vi "zlgcan_demo_CANFDNET_UDP.vi"() -> ()   [LabVIEW 2018]
doc: "适用的设备：CANET-E-U、CANET-2E-U、CANET-4E-U、CANET-8E-U、\nCANET-200T、CANET-100T"
uses:
  zlgcan_demo_CANFDNET_UDP/bin/zlgcan.dll
  zlgcan_demo_CANFDNET_UDP/bin/zlgcan_wrap.dll
  data_type/ZCAN_TransmitFD_Data.ctl
  data_type/ZCAN_Transmit_Data.ctl
panel:
  in  "ZCAN_Transmit_Data":T1
  in  "ZCAN_TransmitFD_Data":T2
  in  "CANFD数据帧数组":T3(array[cluster])
  in  "CAN数据帧数组":T4(array[cluster])
  out "已接收帧数":u32
  out "CAN报文显示":string[][](table)
  out "CANFD报文显示":string[][](table)
  out "error out 2":errorcluster caption="错误输出"
  out "source":string
  in  "开启CAN":bool
  in  "stop":bool
  in  "?":T5(tab)
  in  "CAN卡型号":u32(ring)=49 items=["CANFDNET_800U_UDP"=58, "CANFDNET_400U_UDP"=53, "CANFDNET_100U_UDP"=56, "CANFDNET-200U-UDP"=49]
  in  "索引":u32(ring) items=["0", "1", "2", "3", "4", "5", "6", "7", "8"]
  in  "CAN 通道":u32(ring) items=["0", "1", "2", "3"]
  out "设备句柄":u32
  out "通道句柄":u32
  out "error out":errorcluster caption="状态"
  in  "发送":bool
  in  "ID":u32=18 format="0x%08x"
  in  "帧类型":u32(ring) items=["标准帧", "扩展帧"]
  in  "帧格式":u32(ring) items=["数据帧", "远程帧"]
  in  "发送方式":u32(ring) items=["正常发送", "单次发送", "自发自收", "单次自发自收"]
  in  "协议":u32(ring) items=["CAN", "CANFD"]
  in  "数据输入":string="11 22 33 44 55 66 77 88"
  in  "CANFD加速？":u32(ring) items=["不加速", "加速"]
  out "数据长度":u8=8 max=8
  # "适用的设备：CANFDNET-100U-UDP、CANFDNET-200U-UDP、CANFDNET-400U-UDP、CANFDNET-800U-UDP"
  # "参数设置这里的参数需要到后面板进行设置"
  # "停止程序前，\n请先关闭CAN卡"
  # "当CANFDNET的工作模式为：\n\n1. 客户端（TCP Client）\n\n   LabVIEW 设备型号选择【 CANFDNET-TCP】\n\n   TCP模式选择【服务器 TCP Sever】\n\n   填写电脑本机IP+本地端口。\n\n2. 服务器（TCP Sever）\n\n   LabVIEW 设备型号选择【 CANFDNET-TCP】\n\n   TCP模式选择【客户端 TCP Client】\n\n   填写CANFDNET的 IP +工作端口\n\n3. UDP\n\n   LabVIEW 设备型号选择【 CANFDNET-UDP】\n\n   填写CANFDNET的IP+工作端口+本地端口"
  # "1. 调试运行DEMO前，将bin文件夹下面的kerneldlls文件夹先拷贝至LabView安装目录，\n如 D:\\Program Files (x86)\\National Instruments\\LabVIEW 2018。"
  # "2. 确保电脑有VC++ 2005/2008/2010/2013运行库（对应32，64位），可到微软官网下载。"
  # "3，如果打开设备失败，可能原因：\n（1）没有进行第二步操作；\n（2）已经打开过一次，没有正常关闭的情况下，继续点击“打开设备”，是无法打开的。\n     需要USB重新拔插，LABVIEW重启（全部关闭），然后再“打开设备”。\n (3) 项目路径不能有中文繁体。"
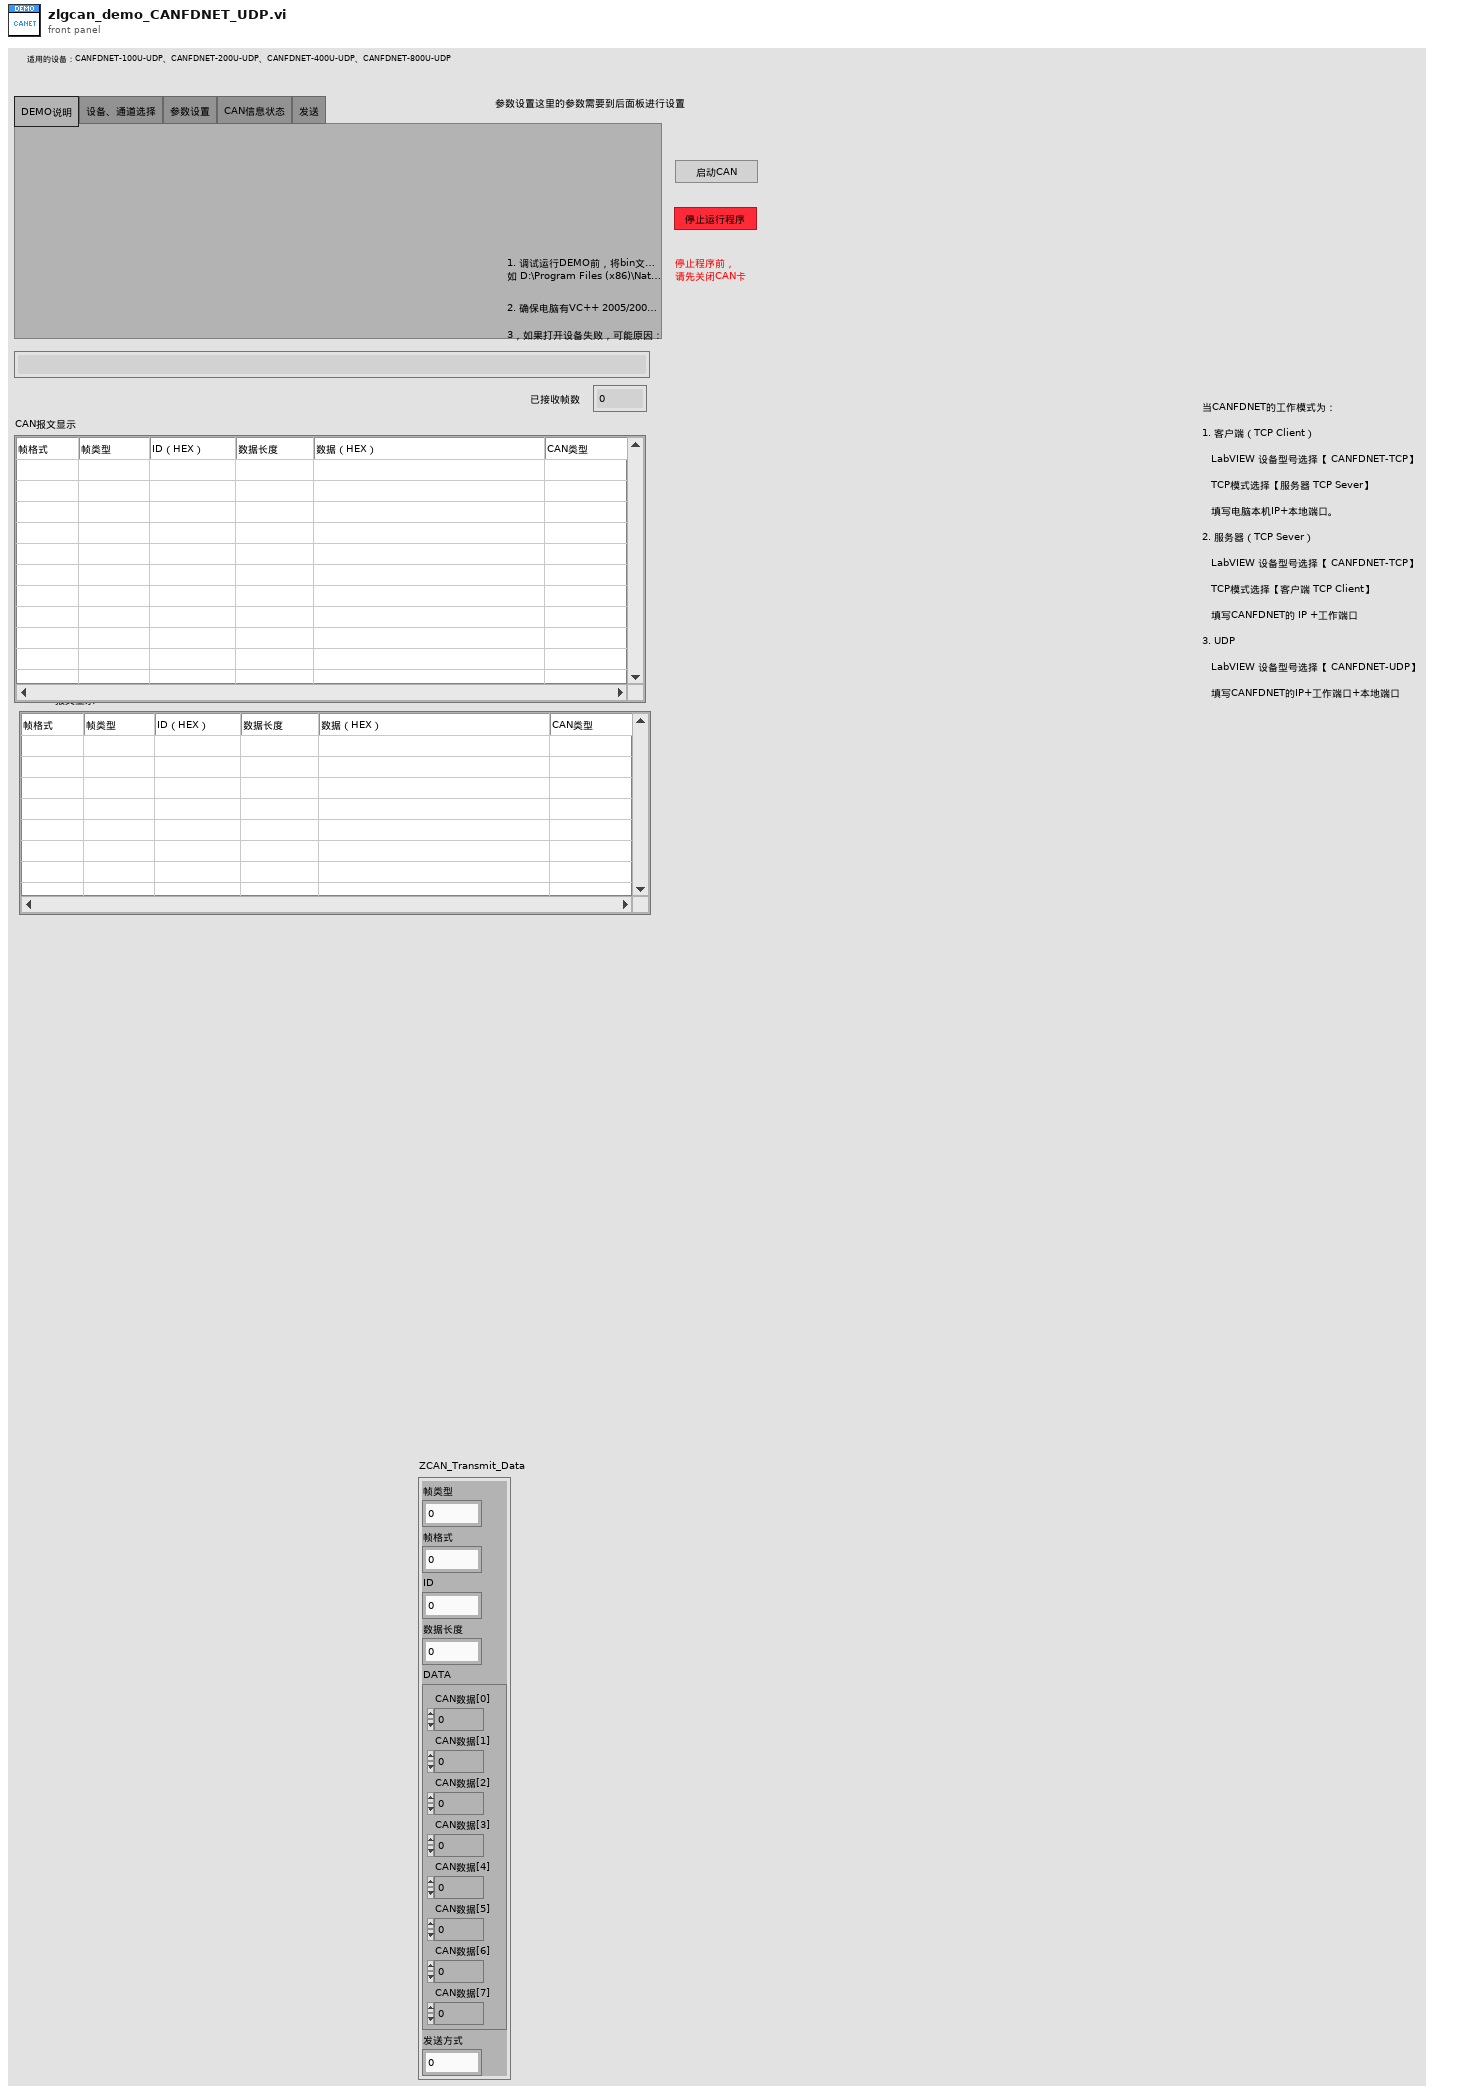
[diagram p1: front panel]
types:
  T1 = typedef "ZCAN_Transmit_Data.ctl" = cluster{"帧类型":u32, "帧格式":u32, "ID":u32, "数据长度":u8, "DATA":cluster{"CAN数据[0]":u8, "CAN数据[1]":u8, "CAN数据[2]":u8, "CAN数据[3]":u8, "CAN数据[4]":u8, "CAN数据[5]":u8, "CAN数据[6]":u8, "CAN数据[7]":u8}, "发送方式":u32}
  T2 = typedef "ZCAN_TransmitFD_Data.ctl" = cluster{"帧类型":u32, "帧格式":u32, "ID":u32, "数据长度":u8, "CANFD加速？":u8, "DATA":cluster{"CAN数据[0]":u8, "CAN数据[1]":u8, "CAN数据[2]":u8, "CAN数据[3]":u8, "CAN数据[4]":u8, "CAN数据[5]":u8, "CAN数据[6]":u8, "CAN数据[7]":u8, "CAN数据[8]":u8, "CAN数据[9]":u8, "CAN数据[10]":u8, "CAN数据[11] ":u8, "CAN数据[12] ":u8, "CAN数据[13] ":u8, "CAN数据[14] ":u8, "CAN数据[15] ":u8, "CAN数据[16]":u8, "CAN数据[17]":u8, "CAN数据[18]":u8, "CAN数据[19]":u8, "CAN数据[20]":u8, "CAN数据[21]":u8, "CAN数据[22]":u8, "CAN数据[23]":u8, "CAN数据[24] ":u8, "CAN数据[25]":u8, "CAN数据[26]":u8, "CAN数据[27]":u8, "CAN数据[28]":u8, "CAN数据[29]":u8, "CAN数据[30]":u8, "CAN数据[31]":u8, "CAN数据[32]":u8, "CAN数据[33]":u8, "CAN数据[34]":u8, "CAN数据[35]":u8, "CAN数据[36]":u8, "CAN数据[37]":u8, "CAN数据[38]":u8, "CAN数据[39]":u8, "CAN数据[40]":u8, "CAN数据[41]":u8, "CAN数据[42]":u8, "CAN数据[43]":u8, "CAN数据[44]":u8, "CAN数据[45]":u8, "CAN数据[46]":u8, "CAN数据[47]":u8, "CAN数据[48]":u8, "CAN数据[49]":u8, "CAN数据[50]":u8, "CAN数据[51]":u8, "CAN数据[52]":u8, "CAN数据[53]":u8, "CAN数据[54]":u8, "CAN数据[55]":u8, "CAN数据[56]":u8, "CAN数据[57]":u8, "CAN数据[58]":u8, "CAN数据[59]":u8, "CAN数据[60]":u8, "CAN数据[61]":u8, "CAN数据[62]":u8, "CAN数据[63]":u8}, "发送方式":u32}
  T3 = cluster{u32, u8, u8, u8, u8, cluster{"[0]":u8, "[1]":u8, "[2]":u8, "[3]":u8, "[4]":u8, "[5]":u8, "[6]":u8, "[7]":u8, "[8]":u8, "[9]":u8, "[10]":u8, "[11]":u8, "[12]":u8, "[13]":u8, "[14]":u8, "[15]":u8, "[16]":u8, "[17]":u8, "[18]":u8, "[19]":u8, "[20]":u8, "[21]":u8, "[22]":u8, "[23]":u8, "[24]":u8, "[25]":u8, "[26]":u8, "[27]":u8, "[28]":u8, "[29]":u8, "[30]":u8, "[31]":u8, "[32]":u8, "[33]":u8, "[34]":u8, "[35]":u8, "[36]":u8, "[37]":u8, "[38]":u8, "[39]":u8, "[40]":u8, "[41]":u8, "[42]":u8, "[43]":u8, "[44]":u8, "[45]":u8, "[46]":u8, "[47]":u8, "[48]":u8, "[49]":u8, "[50]":u8, "[51]":u8, "[52]":u8, "[53]":u8, "[54]":u8, "[55]":u8, "[56]":u8, "[57]":u8, "[58]":u8, "[59]":u8, "[60]":u8, "[61]":u8, "[62]":u8, "[63]":u8}, u64}[]
  T4 = cluster{u32, u8, u8, u8, u8, cluster{"[0]":u8, "[1]":u8, "[2]":u8, "[3]":u8, "[4]":u8, "[5]":u8, "[6]":u8, "[7]":u8}, u64}[]
  T5 = enum32{"DEMO说明", "设备、通道选择", "参数设置", "CAN信息状态", "发送"}
  T6 = cluster{"can_type":u32, "can_type":u32, "can_type":u32, "can_type":u32, "can_type":u8, "can_type":u8, "can_type":u8, "can_type":u8}
  T7 = cluster{"[0]":u32, "[1]":u32, "[2]":u32, "[3]":u32, "[4]":u32, "[5]":u32, "[6]":u32, "[7]":u32, "[8]":u32, "[9]":u32, "[10]":u32, "[11]":u32, "[12]":u32, "[13]":u32, "[14]":u32, "[15]":u32, "[16]":u32, "[17]":u32, "[18]":u32, "[19]":u32, "[20]":u32, "[21]":u32, "[22]":u32, "[23]":u32, "[24]":u32, "[25]":u32, "[26]":u32, "[27]":u32, "[28]":u32, "[29]":u32, "[30]":u32, "[31]":u32, "[32]":u32, "[33]":u32, "[34]":u32, "[35]":u32, "[36]":u32, "[37]":u32, "[38]":u32, "[39]":u32, "[40]":u32, "[41]":u32, "[42]":u32, "[43]":u32, "[44]":u32, "[45]":u32, "[46]":u32, "[47]":u32, "[48]":u32, "[49]":u32, "[50]":u32, "[51]":u32, "[52]":u32, "[53]":u32, "[54]":u32, "[55]":u32, "[56]":u32, "[57]":u32, "[58]":u32, "[59]":u32, "[60]":u32, "[61]":u32, "[62]":u32, "[63]":u32}
  T8 = cluster{"[0]":u32, "[1]":u32, "[2]":u32, "[3]":u32, "[4]":u32, "[5]":u32, "[6]":u32, "[7]":u32}
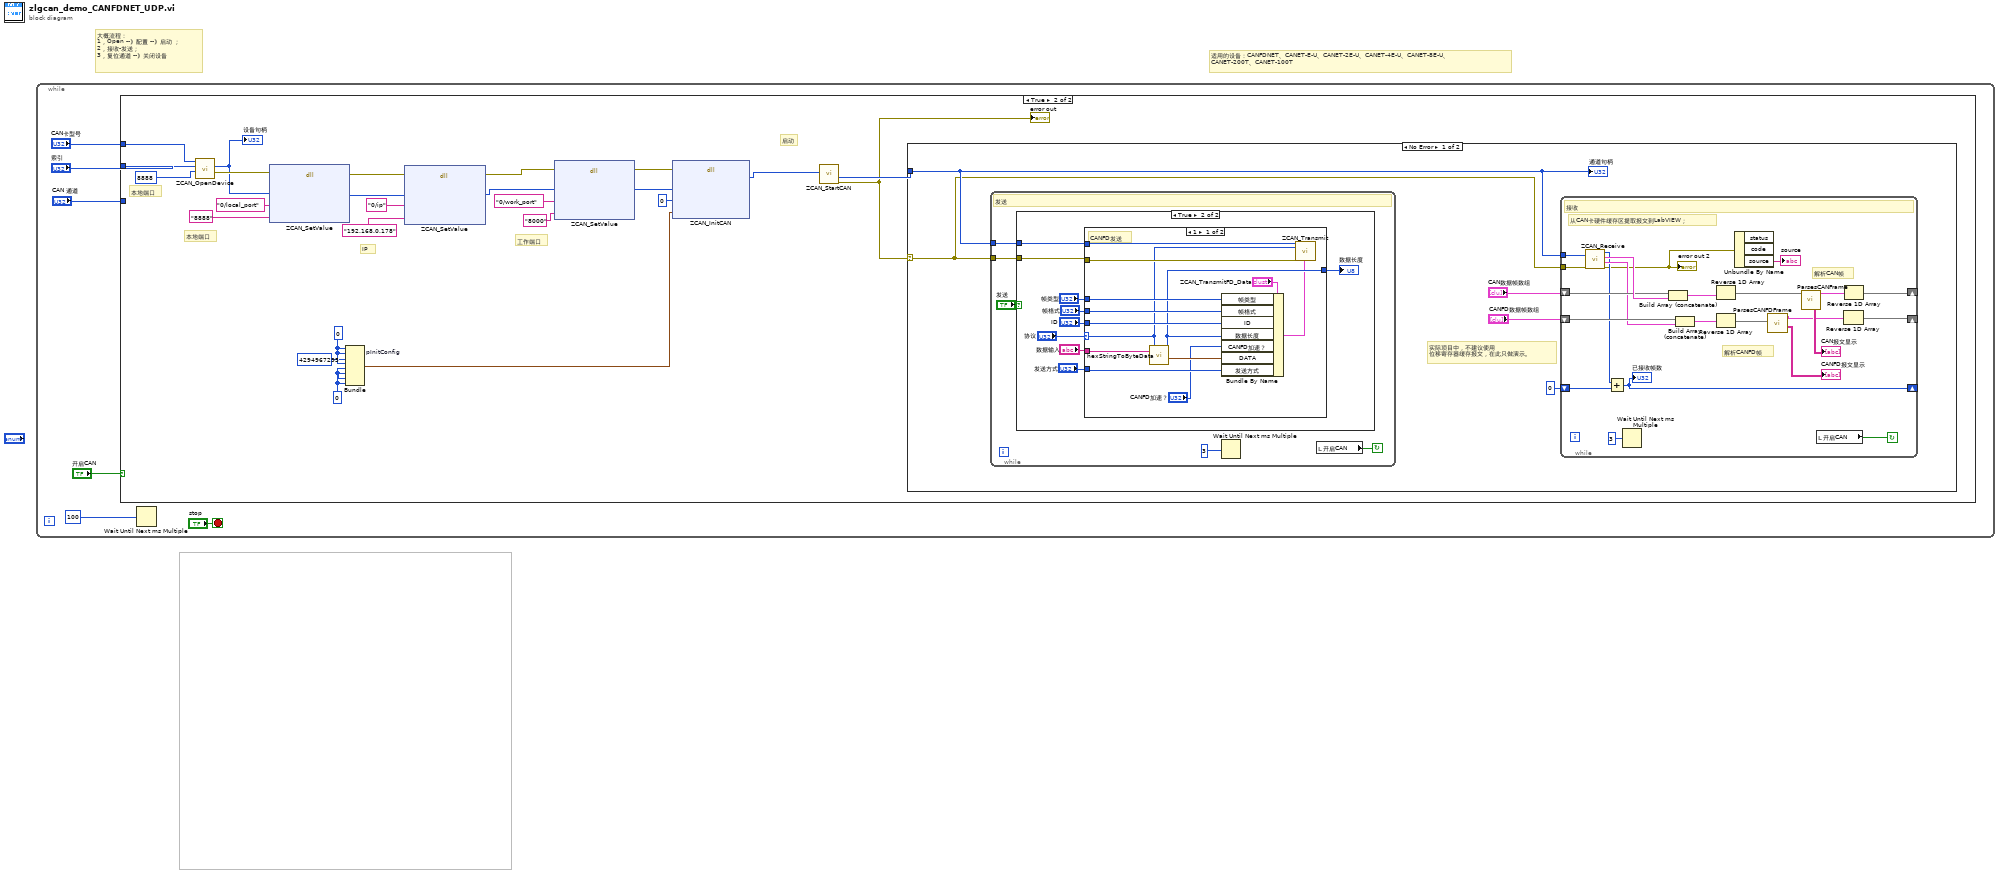
[diagram p0: block diagram]
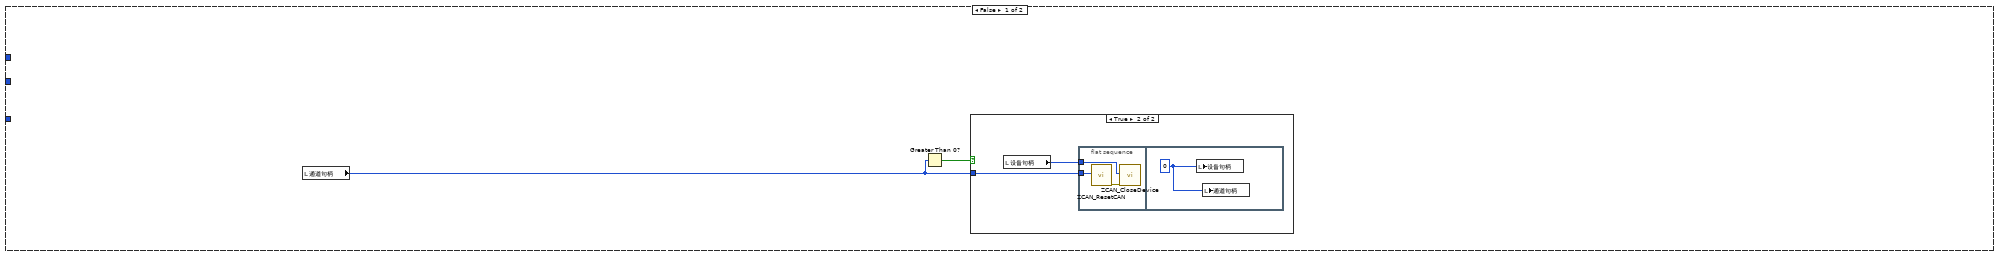
[diagram p2: hidden frame]
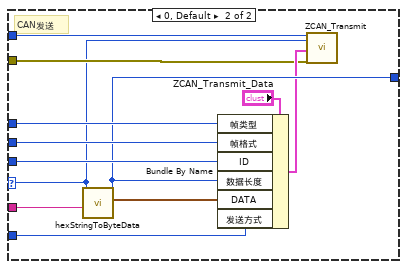
[diagram p5: hidden frame]
diagram:
  # "适用的设备：CANFDNET、CANET-E-U、CANET-2E-U、CANET-4E-U、CANET-8E-U、\nCANET-200T、CANET-100T"
  # "大概流程：\n1，Open --》配置 --》启动 ；\n2，接收-发送；\n3，复位通道 --》关闭设备"
  n1 = while {
    stop <- "stop" stop-if-true
    n2 = case shown="True" "开启CAN" {
      tunnel: "CAN卡型号" -> [_ w35]
      tunnel: "索引" -> [_ w38]
      tunnel: "CAN 通道" -> [_ _]
      frame False {
        # "关闭CAN卡"
        n3 = local read "通道句柄"() -> (w7:u32)
        n4 = Greater Than 0?(x=w7) -> (x > 0?=w8:bool)
        n5 = case shown="True" w8 {
          tunnel: w7 -> [_ w10]
          frame False {
          }
          frame True {
            n6 = local read "设备句柄"() -> (w9:u32)
            n7 = flat-sequence {
              tunnel: w10 -> [w12]
              tunnel: w9 -> [w11]
              frame #0 {
                n8 = call "ZCAN_ResetCAN.vi"("can_handle"=w12) -> ("error out"=w13:errorcluster)  [unwired: 9 in, 1 out]
                n9 = call "ZCAN_CloseDevice.vi"("error in (no error)"=w13, "device_handle"=w11) -> ()  [unwired: 8 in, 2 out]
              }
              frame #1 {
                w14 = u32 0 ("can_index_handle(out)")
                n10 = local write "设备句柄"(w14) -> ()
                n11 = local write "通道句柄"(w14) -> ()
              }
            }
          }
        }
      }
      frame True {
        w16 = u8 0 ("can_type")
        w18 = u32 0 ("can_type")
        # "本地端口"
        # "工作端口"
        # "IP"
        # "启动"
        # "本地端口"
        n12 = call "ZCAN_OpenDevice.vi"("reserved"=8888, "device_index"=w38, "device_type"=w35) -> ("error out"=w24:errorcluster, "DEVICE_HANDLE"=w23:u32)  [unwired: 7 in]
        "设备句柄" <- w23
        n13 = dll-call lib="C:/Users/admin/Desktop/zlgcan_demo_CANFDNET_UDP/bin/zlgcan.dll" fn="ZCAN_SetValue"(error in=w24, "hDev"=w23, "path"="0/local_port", "value"="8888") -> (error out=w26:errorcluster, "hDev"=w31:u32)  [unwired: 5 in, 1 out]
        n14 = Bundle "pInitConfig"("can_type"=w18, "can_type"=w18, "can_type"=u32 4294967295, "can_type"=w18, "can_type"=w16, "can_type"=w16, "can_type"=w16, "can_type"=w16) -> (w19:T6)  [unwired: 1 in]
        n15 = dll-call lib="C:/Users/admin/Desktop/zlgcan_demo_CANFDNET_UDP/bin/zlgcan.dll" fn="ZCAN_SetValue"(error in=w26, "hDev"=w31, "path"="0/ip", "value"="192.168.0.178") -> (error out=w25:errorcluster, "hDev"=w27:u32)  [unwired: 5 in, 1 out]
        n16 = dll-call lib="C:/Users/admin/Desktop/zlgcan_demo_CANFDNET_UDP/bin/zlgcan.dll" fn="ZCAN_SetValue"(error in=w25, "hDev"=w27, "path"="0/work_port", "value"="8000") -> (error out=w22:errorcluster, "hDev"=w21:u32)  [unwired: 5 in, 1 out]
        n17 = dll-call lib="C:/Users/admin/Desktop/zlgcan_demo_CANFDNET_UDP/bin/zlgcan_wrap.dll" fn="ZCAN_InitCAN"(error in=w22, "device_handle"=w21, "can_index"=0, "pInitConfig"=w19) -> ("can_handle"=w15:u32)  [unwired: 5 in, 2 out]
        n18 = call "ZCAN_StartCAN.vi"("can_index_handle"=w15) -> ("error out"=w36:errorcluster, "can_index_handle(out)"=w37:u32)  [unwired: 8 in, 1 out]
        "error out" <- w36
        n19 = case shown="No Error" w36 {
          selector: w36 -> [w40 _]
          tunnel: w37 -> [w41 _]
          frame No Error {
            # "实际项目中，不建议使用\n位移寄存器缓存报文，在此只做演示。"
            n20 = while {
              tunnel: w41 -> [w70]
              tunnel: w40 -> [w68]
              stop <- w69 continue-if-true
              # "发送"
              n21 = case shown="True" "发送" {
                tunnel: w70 -> [_ w73]
                tunnel: w68 -> [_ w74]
                frame False {
                }
                frame True {
                  n22 = case shown="1" "协议" {
                    selector: "协议" -> [w82 w95]
                    tunnel: "帧类型" -> [w93 w105]
                    tunnel: "帧格式" -> [w92 w104]
                    tunnel: "ID" -> [w91 w103]
                    tunnel: "发送方式" -> [w90 w101]
                    tunnel: [w86 w100] -> w76
                    tunnel: "数据输入" -> [w88 w99]
                    tunnel: w74 -> [w85 w97]
                    tunnel: w73 -> [w83 w96]
                    frame 1 {
                      # "CANFD发送"
                      n23 = call "hexStringToByteData.vi"("数据输入"=w88, "协议"=w82) -> ("CANFD_data"=w89:T7, "字节数"=w86:i32)  [unwired: 7 in, 1 out]
                      n24 = Bundle By Name(cluster="ZCAN_TransmitFD_Data", "帧类型"=w93, "帧格式"=w92, "ID"=w91, "数据长度"=w86, "CANFD加速？"="CANFD加速？", "DATA"=w89, "发送方式"=w90) -> (w84:T2)
                      n25 = call "ZCAN_Transmit.vi"("can_index_handle"=w83, "协议"=w82, "error in (no error)"=w85, "ZCAN_TransmitFD_Data"=w84) -> ()  [unwired: 15 in, 1 out]
                    }
                    frame 0, Default {
                      # "CAN发送"
                      n26 = call "hexStringToByteData.vi"("数据输入"=w99, "协议"=w95) -> ("CAN_data"=w102:T8, "字节数"=w100:i32)  [unwired: 7 in, 1 out]
                      n27 = Bundle By Name(cluster="ZCAN_Transmit_Data", "帧类型"=w105, "帧格式"=w104, "ID"=w103, "数据长度"=w100, "DATA"=w102, "发送方式"=w101) -> (w98:T1)
                      n28 = call "ZCAN_Transmit.vi"("can_index_handle"=w96, "协议"=w95, "ZCAN_Transmit_Data"=w98, "error in (no error)"=w97) -> ()  [unwired: 15 in, 1 out]
                    }
                  }
                  "数据长度" <- w76
                }
              }
              n29 = Wait Until Next ms Multiple(millisecond multiple=u32 3) -> ()  [unwired: 1 out]
              n30 = local read "开启CAN"() -> (w69:bool)
            }
            n31 = while {
              tunnel: w40 -> [w65]
              tunnel: w41 -> [w64]
              shift-right: [w66] -> _
              shift-left: 0 -> [w52]
              shift-right: [w56] -> _
              shift-left: "CAN数据帧数组" -> [w62]
              shift-right: [w54] -> _
              shift-left: "CANFD数据帧数组" -> [w60]
              stop <- w45 continue-if-true
              # "从CAN卡硬件缓存区提取报文到LabVIEW；"
              # "解析CANFD帧"
              # "解析CAN帧"
              # "接收"
              n32 = call "ZCAN_Receive.vi"("error in (no error)"=w65, "can_handle"=w64) -> ("error out"=w46:errorcluster, "CANFD数据帧数组"=w59:T3, "CAN数据帧数组"=w63:T4, "Receive_Num"=w53:u32)  [unwired: 2 in]
              "error out 2" <- w46
              n33 = Add(x=w53, y=w52) -> (x+y=w66:u32)
              "已接收帧数" <- w66
              n34 = Wait Until Next ms Multiple(millisecond multiple=u32 3) -> ()  [unwired: 1 out]
              n35 = Build Array (concatenate)(w62, w63) -> (w61:T4)
              n36 = Build Array (concatenate)(w60, w59) -> (w58:T3)
              n37 = Reverse 1D Array(array=w61) -> (reversed array=w55:T4)
              n38 = Reverse 1D Array(array=w58) -> (reversed array=w50:T3)
              n39 = Unbundle By Name(w46) -> ("source"=→"source":string)  [unwired: 2 out]
              n40 = call "ParsesCANFDFrame.vi"("CANFD数据帧数组"=w50) -> ("CANFD报文显示"=→"CANFD报文显示":string[][], "CANFD数据帧数组(out)"=w49:T3)  [unwired: 9 in]
              n41 = call "ParsesCANFrame.vi"("CAN数据帧数组"=w55) -> ("CAN数据帧数组(out)"=w57:T4, "CAN报文显示"=→"CAN报文显示":string[][])  [unwired: 9 in]
              n42 = local read "开启CAN"() -> (w45:bool)
              n43 = Reverse 1D Array(array=w49) -> (reversed array=w54:T3)
              n44 = Reverse 1D Array(array=w57) -> (reversed array=w56:T4)
            }
            "通道句柄" <- w41
          }
          frame Error {
          }
        }
      }
    }
    n45 = Wait Until Next ms Multiple(millisecond multiple=u32 100) -> ()  [unwired: 1 out]
  }
